vi "CRYRename Channel Info.vi"(9 "Channel Info In":T1[](array[typedef]) {"Coupling" items=["Default"=-1, "RSE"=10083, "NRSE"=10078, "Differential"=10106, "Pseudodifferential"=12529]; "term config" items=["Default"=-1, "RSE"=10083, "NRSE"=10078, "Differential"=10106, "Pseudodifferential"=12529]; "Anti-aliasing Factor (%fs)" format="%.2f"}, 10 "Channel Name":string, 11 "Selected Index":u16) -> (1 "Channel Info Out":T1[](array[typedef]) {"Coupling" items=["Default"=-1, "RSE"=10083, "NRSE"=10078, "Differential"=10106, "Pseudodifferential"=12529]; "term config" items=["Default"=-1, "RSE"=10083, "NRSE"=10078, "Differential"=10106, "Pseudodifferential"=12529]; "Anti-aliasing Factor (%fs)" format="%.2f"}, 2 "Name Array":string[](array[string]), 3 "New Index":u16)   [LabVIEW 2013]
uses:
  Typedef Control/CRYHardware Channel Info.ctl
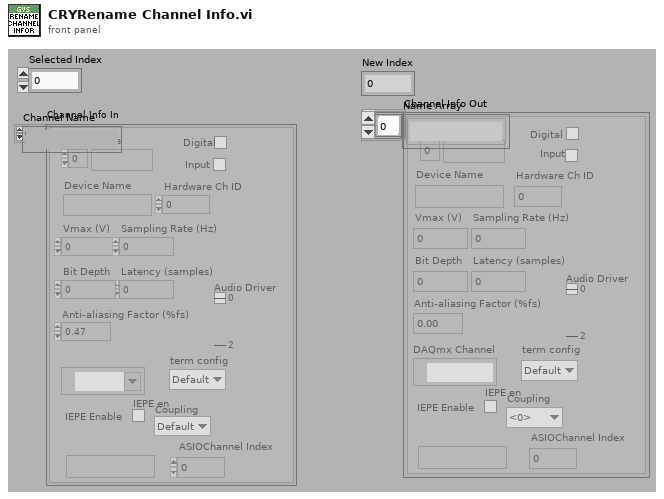
[diagram p1: front panel]
types:
  T1 = typedef "CRYHardware Channel Info.ctl" = cluster{"ID":i32, "Name":string, "Digital":bool, "Input":bool, "Device Name":string, "Hardware Ch ID":u8, "Vmax (V)":dbl, "Latency (samples)":dbl, "Sampling Rate (Hz)":u32, "Bit Depth":u32, "Anti-aliasing Factor (%fs)":sgl, "DAQmx Channel":tag, "term config":i32, "Coupling":i32, "IEPE en":bool, "ASIOChannel Name":string, "Audio Driver":u16, "ASIOChannel Index":u8}
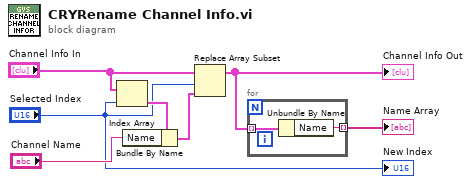
[diagram p0: block diagram]
diagram:
  n1 = Index Array(array="Channel Info In", index="Selected Index") -> (element=w7:T1)
  n2 = Bundle By Name(cluster=w7, "Name"="Channel Name") -> (w6:T1)
  n3 = Replace Array Subset(array="Channel Info In", new element=w6, index="Selected Index") -> (w3:T1[])
  "Channel Info Out" <- w3
  n4 = for {
    tunnel: w3 -> [w9] mode=indexing
    tunnel: [w8] -> w2 mode=indexing
    n5 = Unbundle By Name(w9) -> ("Name"=w8:string)
  }
  "Name Array" <- w2
  "New Index" <- "Selected Index"
